vi "Show Dialog.vi"(8 "error in (no error)":errorcluster, 10 "User VI Ref":refnum<vi>, 11 "Error Cluster":errorcluster) -> (0 "error out":errorcluster)   [LabVIEW 2020, in "Explain Error Improved Dialog.lvlib" / "Explain Error Improved Dialog.lvclass"]
uses:
  <resource>/plugins/PopupMenus/edit time panel and diagram/Explain Error (Improved)/Explain Error Improved Dialog/Explain Error Improved Dialog/Explain Error Improved Dialog.lvclass
  C:/Program Files/National Instruments/LabVIEW 2020/vi.lib/ActorFramework/Actor/Actor.lvclass
  <resource>/plugins/PopupMenus/edit time panel and diagram/Explain Error (Improved)/Explain Error Improved Dialog/Explain Error Improved Dialog/Explain Error Improved Dialog.lvclass/Explain Error Improved Dialog.ctl
  <vilib>/ActorFramework/Actor/Actor.lvclass
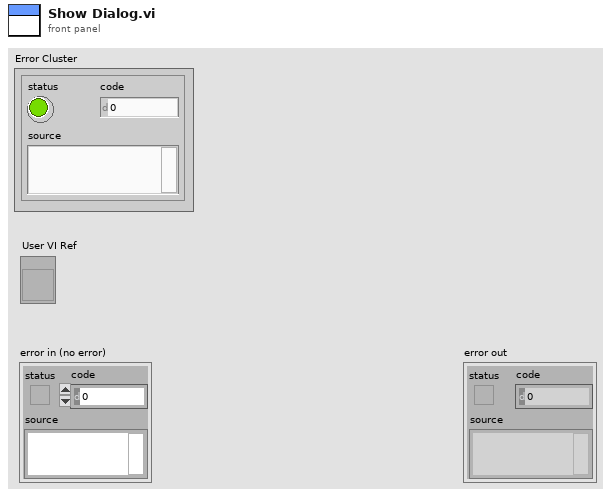
[diagram p1: front panel]
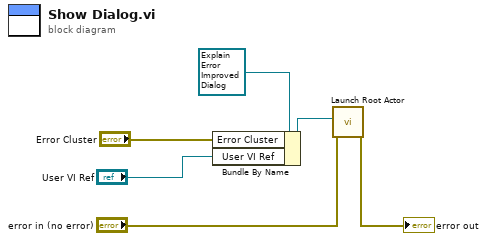
[diagram p0: block diagram]
diagram:
  n1 = Bundle By Name(cluster=refnum<class "Explain Error Improved Dialog.lvclass"> refnum ("Explain Error Improved Dialog.lvlib:Explain Error Improved Dialog.lvclass"), "Error Cluster"="Error Cluster", "User VI Ref"="User VI Ref") -> (w5:refnum<class "Explain Error Improved Dialog.lvclass">)
  n2 = call <vilib>:"Launch Root Actor.vi"("error in (no error)"="error in (no error)", "Actor"=w5) -> ("error out"=→"error out":errorcluster)  [unwired: 8 in, 1 out]
